vi "_f_IEEE754format.vi"(8 "error in (no error)":errorcluster, 9 "String":string="459CFFAE") -> (0 "error out":errorcluster, 1 "Number":sgl=92.92 format="%.2f")   [LabVIEW 2013]
panel:
  # "Binary Storage Format to SGL"
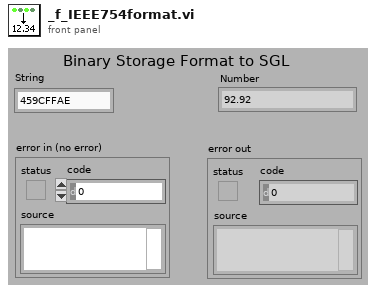
[diagram p1: front panel]
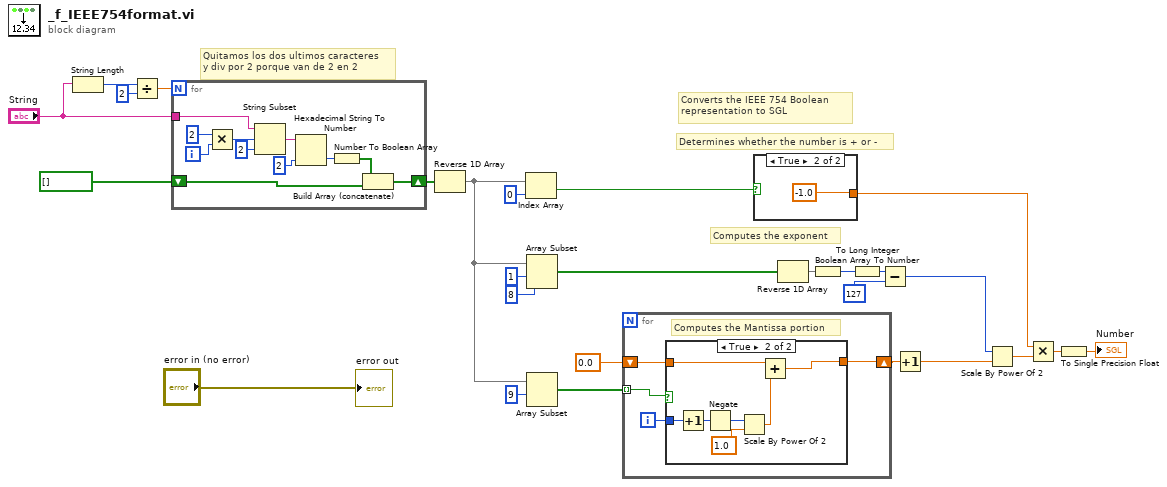
[diagram p0: block diagram]
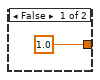
[diagram p2: hidden frame]
diagram:
  # "Converts the IEEE 754 Boolean \nrepresentation to SGL"
  # "Computes the exponent"
  # "Determines whether the number is + or -"
  # "Quitamos los dos ultimos caracteres\ny div por 2 porque van de 2 en 2"
  n1 = String Length(string="String") -> (length=w22:i32)
  n2 = Divide(x=w22, y=2) -> (x/y=w26:dbl)
  n3 = for {
    N: w26 -> [_]
    tunnel: "String" -> [w34]
    shift-right: [w29] -> w23
    shift-left: bool[] [] -> [w28]
    i -> [w36]
    n4 = Multiply(x=2 ("length (rest)"), y=w36) -> (x*y=w35:i32)
    n5 = String Subset(string=w34, offset (0)=w35, length (rest)=2 ("length (rest)")) -> (substring=w33:string)
    n6 = Hexadecimal String To Number(string=w33, default (0uL)=u8 2 ("length (rest)")) -> (number=w31:u8)  [unwired: 1 in, 1 out]
    n7 = Number To Boolean Array(number=w31) -> (Boolean array=w30:bool[])
    n8 = Build Array (concatenate)(w30, w28) -> (w29:bool[])
  }
  n9 = Reverse 1D Array(array=w23) -> (reversed array=w21:bool[])
  n10 = Index Array(array=w21, index=0) -> (element=w2:bool)
  n11 = Array Subset(array=w21, index=1, length=8) -> (w5:bool[])
  n12 = Array Subset(array=w21, index=9) -> (w4:bool[])  [unwired: 1 in]
  n13 = for {
    tunnel: w4 -> [w42] mode=indexing
    shift-right: [w39] -> w16
    shift-left: 0.0 -> [w40]
    i -> [w41]
    # "Computes the Mantissa portion"
    n14 = case shown="True" w42 {
      tunnel: w41 -> [_ w50]
      tunnel: w40 -> [w43 w46]
      tunnel: [w43 w44] -> w39
      frame False {
      }
      frame True {
        n15 = Increment(x=w50) -> (x+1=w49:i32)
        n16 = Negate(x=w49) -> (-x=w48:i32)
        n17 = Scale By Power Of 2(n=w48, x=1.0) -> (x*2^n=w45:dbl)
        n18 = Add(x=w46, y=w45) -> (x+y=w44:dbl)
      }
    }
  }
  n19 = case shown="True" w2 {
    tunnel: [1.0 -1.0] -> w10
    frame False {
    }
    frame True {
    }
  }
  n20 = Reverse 1D Array(array=w5) -> (reversed array=w12:bool[])
  n21 = Boolean Array To Number(Boolean array=w12) -> (number=w8:u32)
  n22 = To Long Integer(number=w8) -> (32bit integer=w7:i32)
  n23 = Subtract(x=w7, y=127) -> (x-y=w9:i32)
  n24 = Increment(x=w16) -> (x+1=w14:dbl)
  n25 = Scale By Power Of 2(n=w9, x=w14) -> (x*2^n=w13:dbl)
  n26 = Multiply(x=w10, y=w13) -> (x*y=w11:dbl)
  n27 = To Single Precision Float(number=w11) -> (single precision float=→"Number":sgl)
  "error out" <- "error in (no error)"
